vi "WSVCAP SHL Host TL RFFE Write Cycle - Multiple DUTs - Common Data.vi"(0 "Data Out (Cycle Commands)":string[](array[string]), 5 "Post Command Delay":dbl[](array[numeric]) format="%#.0p s", 11 "error in":errorcluster, 12 "FPGA":T1, 13 "DUT Mask (All)":bool[](array[boolean])=[TRUE, TRUE, TRUE, TRUE, TRUE, TRUE, TRUE, TRUE, TRUE, TRUE, TRUE, TRUE, TRUE, TRUE, TRUE, TRUE, TRUE, TRUE, TRUE, TRUE, TRUE, TRUE, TRUE, TRUE, TRUE, TRUE, TRUE, TRUE, TRUE, TRUE, TRUE, TRUE, TRUE, TRUE, TRUE, TRUE], 14 "Log (T)":bool=TRUE) -> (15 "error out":errorcluster)   [LabVIEW 2012]
uses:
  Type Defs/WSVCAP SHL I2C FPGA Enum.ctl
panel:
  out "Socket Mask":u64=1 format="%02x"
  out "RFFE Data Out [U8]":u8[][](array[numeric]) format="%02x"
  # "DUT 01"
  # "DUT 02"
  # "DUT 03"
  # "DUT 04"
  # "DUT 05"
  # "DUT 06"
  # "DUT 07"
  # "DUT 08"
  # "DUT 09"
  # "DUT 10"
  # "DUT 11"
  # "DUT 12"
  # "DUT 13"
  # "DUT 14"
  # "DUT 15"
  # "DUT 16"
  # "DUT 17"
  # "DUT 18"
  # "DUT 19"
  # "DUT 20"
  # "DUT 21"
  # "DUT 22"
  # "DUT 23"
  # "DUT 24"
  # "DUT 25"
  # "DUT 26"
  # "DUT 27"
  # "DUT 28"
  # "DUT 29"
  # "DUT 30"
  # "DUT 31"
  # "DUT 32"
  # "DUT 33"
  # "DUT 34"
  # "DUT 35"
  # "DUT 36"
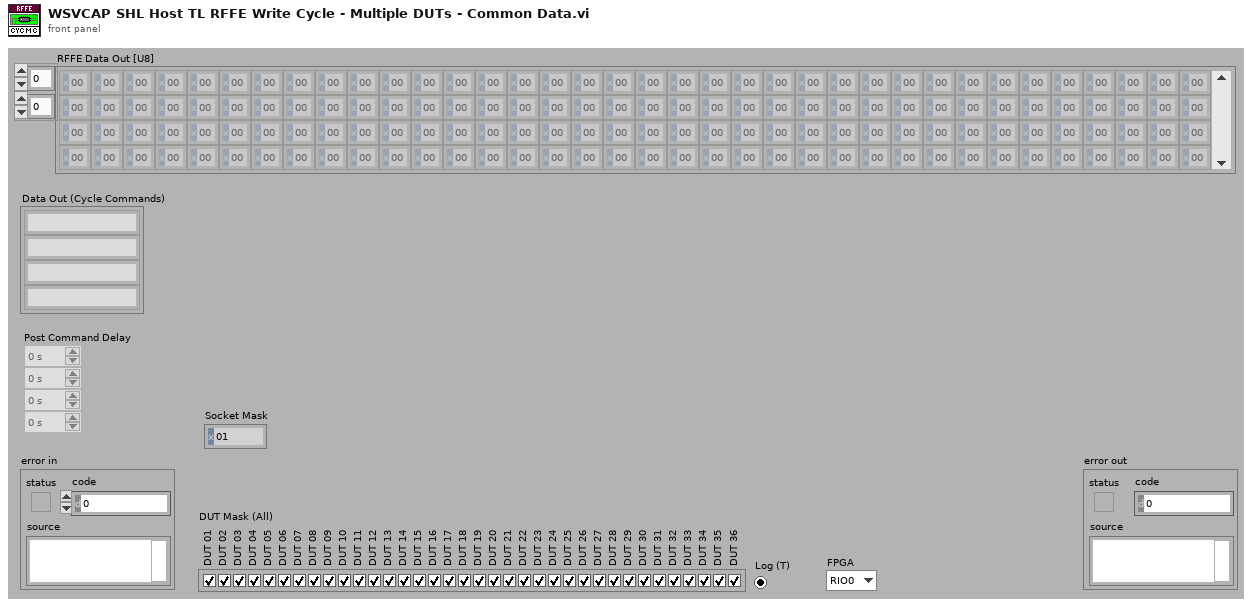
[diagram p1: front panel]
types:
  T1 = typedef "WSVCAP SHL I2C FPGA Enum.ctl" = enum16{"RIO0", "RIO1"}
  T2 = typedef "WSVCAP SHL Core System Cluster.ctl" = cluster{"Settings":T3, "FPGA Resource":tag, "Online":bool, "I2C Wait Ticks":u32, "SPI Wait Ticks":u32, "RFFE Wait Ticks":u32, "FPGA VI Reference (FPGA Mode)":T4, "FPGA VI Reference (Sim Mode)":refnum<vi>}
  T3 = typedef "WSVCAP SHL I2C Settings Cluster.ctl" = cluster{"I2C Slave Address":u8, "I2C Clock Rate (Hz)":dbl, "SPI Clock Rate (Hz)":dbl, "RFFE Slave Address":u8, "RFFE Clock Rate (Hz)":dbl, "Simulate FPGA":bool, "C1 Cap DAC Default":u8, "C2 Cap DAC Default":u8, "C3 Cap DAC Default":u8}
  T4 = typedef "WSVCAP SHL FPGA VI Reference.ctl" = refnum<k20>
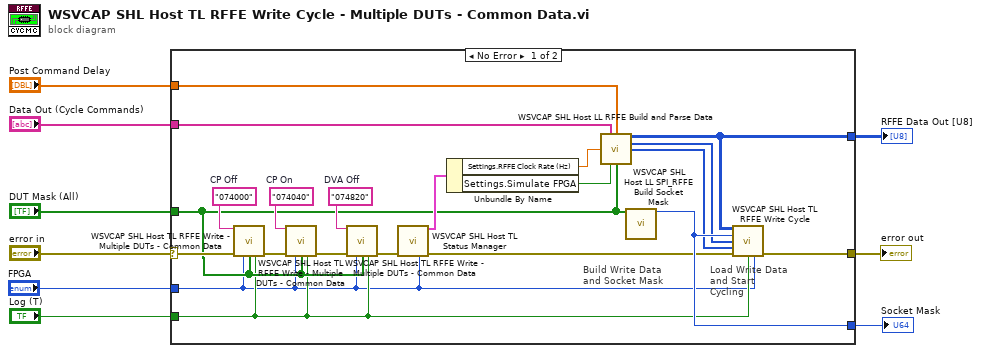
[diagram p0: block diagram]
diagram:
  n1 = case shown="No Error" "error in" {
    selector: "error in" -> [w18 _]
    tunnel: [w30 _] -> w9
    tunnel: [w29 _] -> w7
    tunnel: [w28 _] -> w6
    tunnel: "DUT Mask (All)" -> [w12 _]
    tunnel: "Post Command Delay" -> [w27 _]
    tunnel: "Data Out (Cycle Commands)" -> [w26 _]
    tunnel: "Log (T)" -> [w11 _]
    tunnel: "FPGA" -> [w10 _]
    frame No Error {
      w13 = "074820"  # DVA Off
      w14 = "074040"  # CP On
      w15 = "074000"  # CP Off
      # "Load Write Data and Start Cycling"
      # "Build Write Data and Socket Mask"
      n2 = call "WSVCAP SHL Host TL RFFE Write - Multiple DUTs - Common Data.vi"("Data Out"=w15, "error in"=w18, "FPGA"=w10, "DUT Mask (All)"=w12, "Log (T)"=w11) -> ("error out"=w19:errorcluster)  [unwired: 10 in]
      n3 = call "WSVCAP SHL Host TL RFFE Write - Multiple DUTs - Common Data.vi"("Data Out"=w14, "error in"=w19, "FPGA"=w10, "DUT Mask (All)"=w12, "Log (T)"=w11) -> ("error out"=w17:errorcluster)  [unwired: 10 in]
      n4 = call "WSVCAP SHL Host TL RFFE Write - Multiple DUTs - Common Data.vi"("Data Out"=w13, "error in"=w17, "FPGA"=w10, "DUT Mask (All)"=w12, "Log (T)"=w11) -> ("error out"=w16:errorcluster)  [unwired: 10 in]
      n5 = call "WSVCAP SHL Host TL Status Manager.vi"("error in"=w16, "FPGA"=w10) -> ("System Out"=w25:T2, "error out"=w24:errorcluster)  [unwired: 12 in]
      n6 = Unbundle By Name(w25) -> ("Settings.RFFE Clock Rate (Hz)"=w20:dbl, "Settings.Simulate FPGA"=w23:bool)
      n7 = call "WSVCAP SHL Host LL RFFE Build and Parse Data.vi"("Data Out (Cycle Commands)"=w26, "Post Command Delay"=w27, "Clock Rate (Hz) (Cycle Only)"=w20, "Simulate FPGA (Cycle Only)"=w23, "DUT Mask (All)"=w12) -> ("RFFE Data Out [U8]"=w29:u8[][], "CMD Lengths (Bits)"=w22:u8[], "CMD Delays (Ticks)"=w21:u32[])  [unwired: 7 in, 1 out]
      n8 = call "WSVCAP SHL Host LL SPI_RFFE Build Socket Mask.vi"("DUT Mask"=w12) -> ("Socket Mask [U64]"=w28:u64)  [unwired: 14 in]
      n9 = call "WSVCAP SHL Host TL RFFE Write Cycle.vi"("RFFE Data Out"=w29, "Socket Mask"=w28, "Cycle CMD Lengths (bits)"=w22, "Cycle CMD Delay (ticks)"=w21, "error in"=w24, "Log (T)"=w11, "FPGA"=w10) -> ("error out"=w30:errorcluster)  [unwired: 8 in]
    }
    frame Error {
    }
  }
  "error out" <- w9
  "RFFE Data Out [U8]" <- w7
  "Socket Mask" <- w6
